vi "UP+Left.vi"() -> ()   [LabVIEW 2013]
uses:
  <vilib>/event_ctls.llb/eventvkey.ctl
panel:
  out "Both":bool
  # "Boolean turns TRUE if both\nUP and LEFT is held down\nFALSE otherwise."
  # "http://forums.ni.com/t5/LabVIEW/Simultaneous-keys-for-quot-Key-Repeat-quot-event/m-p/1269402#M530500"
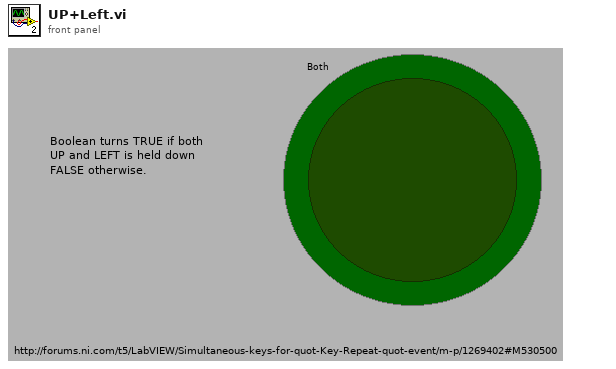
[diagram p1: front panel]
types:
  T1 = typedef "eventvkey.ctl" = enum16{"ASCII", "Enter", "Return", "Shift", "Ctrl", "Alt", "Cmd", "Opt", "Caps", "NumLock", "Clear", "Break", "Up", "Down", "Left", "Right", "Insert", "Delete", "Home", "End", "PageUp", "PageDown", "Escape", "Help", "Pause", "ScrollLock", "F1", "F2", "F3", "F4", "F5", "F6", "F7", "F8", "F9", "F10", "F11", "F12", "F13", "F14", "F15", "F16", "F17", "F18", "F19", "F20", "F21", "F22", "F23", "F24", "Play", "VolumeUp", "VolumeDown", "Mute", "Two Byte Char"}
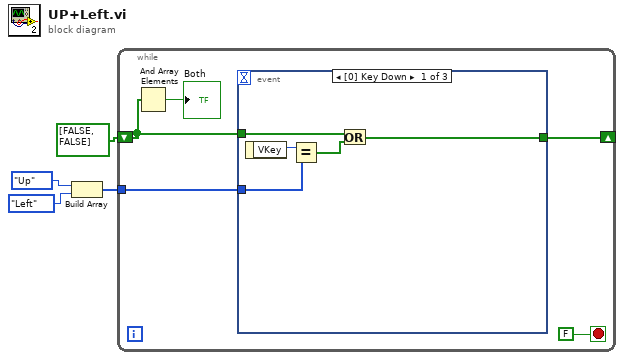
[diagram p0: block diagram]
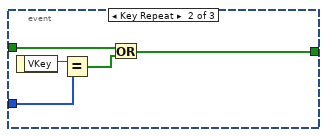
[diagram p2: hidden frame]
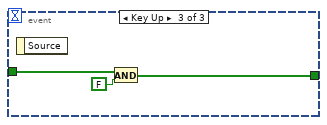
[diagram p3: hidden frame]
diagram:
  n1 = Build Array(eventvkey."Up" ("VKey"), eventvkey."Left" ("VKey")) -> (w3:T1[])
  n2 = while {
    tunnel: w3 -> [w8]
    shift-right: [w7] -> _
    shift-left: bool[] [FALSE, FALSE] -> [w6]
    stop <- FALSE stop-if-true
    n3 = And Array Elements(Boolean array=w6) -> (logical AND=→"Both":bool)
    n4 = event shown="[0] Key Down" {
      selector: _ -> [_ _ _]
      dyn-events: _ -> [_ _ _]
      timeout: _ -> [_ _ _]
      tunnel: w8 -> [w13 w18 _]
      tunnel: w6 -> [w11 w16 w22]
      tunnel: [w10 w15 w21] -> w7
      event Key Down {
        n5 = event-data() -> ("VKey"=w14:T1)  [unwired: 1 in]
        n6 = Equal?(x=w14, y=w13) -> (x = y?=w12:bool[])
        n7 = Or(x=w11, y=w12) -> (x .or. y?=w10:bool[])
      }
      event Key Repeat {
        n8 = event-data() -> ("VKey"=w19:T1)  [unwired: 1 in]
        n9 = Equal?(x=w19, y=w18) -> (x = y?=w17:bool[])
        n10 = Or(x=w16, y=w17) -> (x .or. y?=w15:bool[])
      }
      event Key Up {
        n11 = event-data() -> ()  [unwired: 1 in, 1 out]
        n12 = And(x=w22, y=FALSE) -> (x .and. y?=w21:bool[])
      }
    }
  }
